vi "EventServer_GetClientList.vi"(8 "error in (no error)":errorcluster) -> (0 "error out":errorcluster, 3 "Client List":string[](array[string]))   [LabVIEW 2018]
uses:
  Modules/EventClient_ObjectReference.ctl
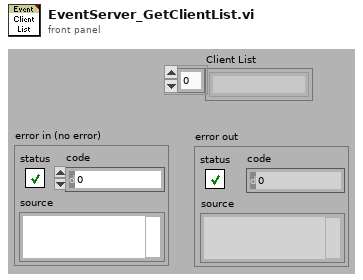
[diagram p1: front panel]
types:
  T1 = typedef "EventClient_ObjectReference.ctl" = refnum<k1>
  T2 = cluster{"Client":refnum<queue>, "Sub Events":string[], "PrvData":variant, "MyName":string}
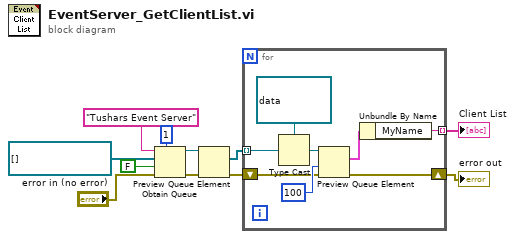
[diagram p0: block diagram]
diagram:
  w7 = T1[] [] items=["EventClient"]
  n1 = Obtain Queue(max queue size (-1, unlimited)=1, name (unnamed)="Tushars Event Server", element data type=w7, create if not found? (T)=FALSE, error in (no error)="error in (no error)") -> (queue out=w9:refnum<queue>, error out=w10:errorcluster)  [unwired: 1 out]
  n2 = Preview Queue Element(queue=w9, error in (no error)=w10) -> (element=w6:T1[], error out=w5:errorcluster)  [unwired: 3 out]
  n3 = for {
    tunnel: w6 -> [w19] mode=indexing
    shift-right: [w13] -> w4
    shift-left: w5 -> [w15]
    tunnel: [w12] -> w1 mode=indexing
    n4 = Type Cast(type=refnum<queue> refnum ("queue out"), x=w19) -> (*(type *) &x=w18:refnum<queue>)
    n5 = Preview Queue Element(queue=w18, timeout in ms (-1)=100, error in (no error)=w15) -> (element=w17:T2, error out=w13:errorcluster)  [unwired: 2 out]
    n6 = Unbundle By Name(w17) -> ("MyName"=w12:string)
  }
  "error out" <- w4
  "Client List" <- w1
